vi "Elevator - State Exit.vi"(8 "error in (no error)":errorcluster, 11 "View Model":T1) -> (0 "error out":errorcluster, 3 "View Model":T1)   [LabVIEW 2017]
doc: "Perform actions before finish a specific state."
uses:
  View Model/Controls/View Model.ctl
  Configuration/Controls/Config Model.ctl
  Configuration/Controls/Config Data.ctl
  Error Handler/Controls/Error Model.ctl
  Error Handler/Controls/Error Data.ctl
  Error Handler/Controls/Error Type.ctl
  View Model/Controls/Shared Model.ctl
  Controls/Elevator Model.ctl
  Controls/Elevator Location.ctl
  Controls/Elevator CMD Data.ctl
  Controls/Elevator Commands.ctl
  Controls/Elevator Overhead.ctl
  Controls/Elevator States.ctl
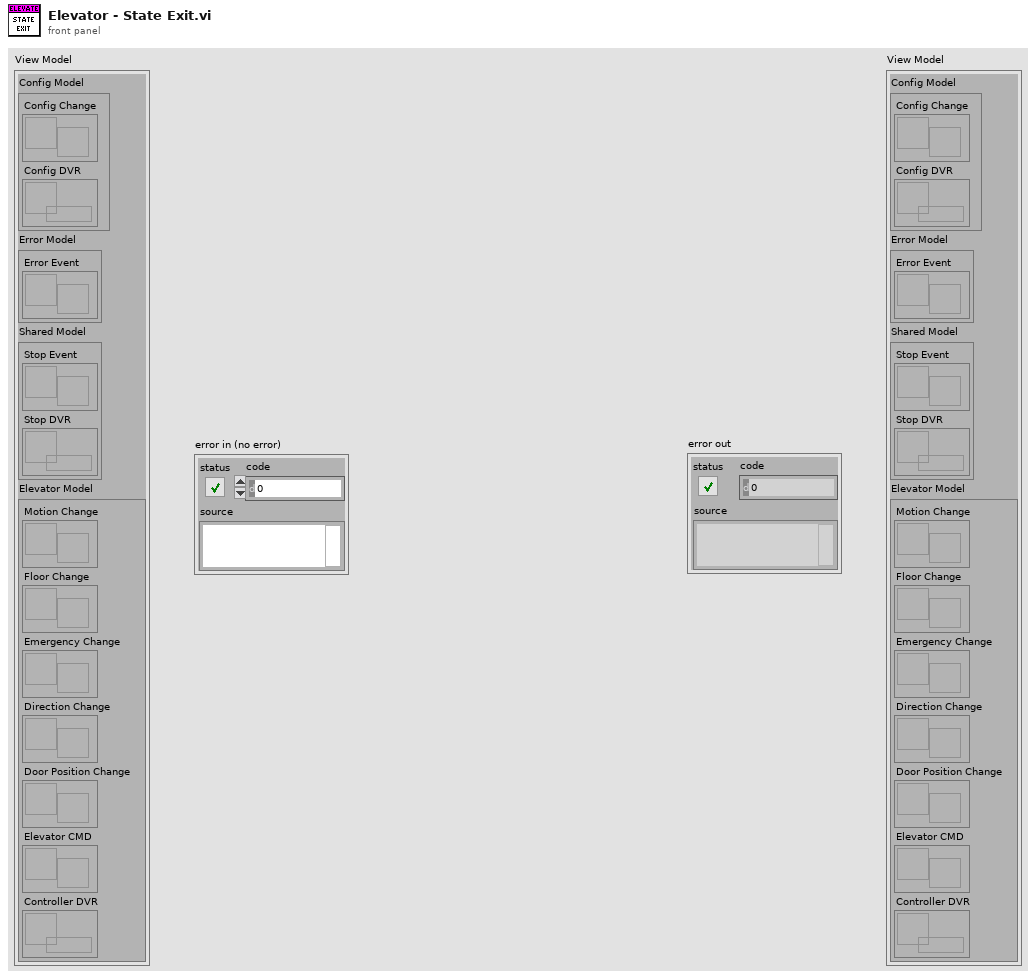
[diagram p1: front panel]
types:
  T1 = typedef "View Model.ctl" = cluster{"Config Model":T2, "Error Model":T3, "Shared Model":T4, "Elevator Model":T5}
  T2 = typedef "Config Model.ctl" = cluster{"Config Change":refnum<user-event>, "Config DVR":refnum<data-value>}
  T3 = typedef "Error Model.ctl" = cluster{"Error Event":refnum<user-event>}
  T4 = typedef "Shared Model.ctl" = cluster{"Stop Event":refnum<user-event>, "Stop DVR":refnum<data-value>}
  T5 = typedef "Elevator Model.ctl" = cluster{"Motion Change":refnum<user-event>, "Floor Change":refnum<user-event>, "Emergency Change":refnum<user-event>, "Direction Change":refnum<user-event>, "Door Position Change":refnum<user-event>, "Elevator CMD":refnum<user-event>, "Controller DVR":refnum<data-value>}
  T6 = typedef "Elevator States.ctl" = enum16{"Initial", "Wait for 1st Request", "Start and Move", "Analysis", "Continue Travel", "Stop at Floor", "Open and Close Door", "No Request", "Emergency", "Terminate"}
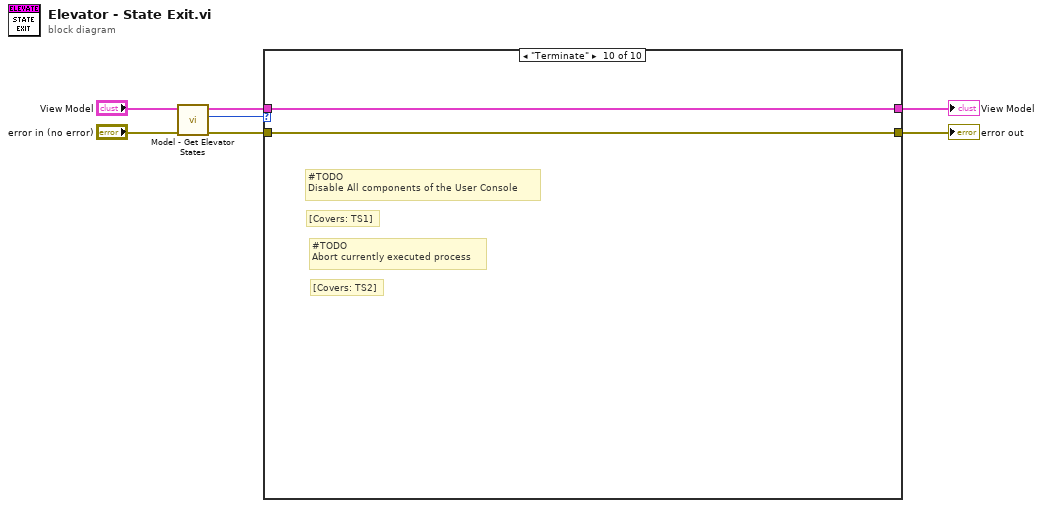
[diagram p0: block diagram]
diagram:
  n1 = call "Model - Get Elevator States.vi"("error in (no error)"="error in (no error)", "View Model"="View Model") -> ("error out"=w3:errorcluster, "Elevator State"=w5:T6, "View Model"=w4:T1)  [unwired: 6 in, 1 out]
  n2 = case shown="\"Terminate\"" w5 {
    tunnel: w4 -> [w9 w11 w13 w15 w17 w19 w21 w23 w25 w27]
    tunnel: w3 -> [w8 w10 w12 w14 w16 w18 w20 w22 w24 w26]
    tunnel: [w9 w11 w13 w15 w17 w19 w21 w23 w25 w27] -> w2
    tunnel: [w8 w10 w12 w14 w16 w18 w20 w22 w24 w26] -> w1
    frame "Initial", Default {
    }
    frame "Wait for 1st Request" {
    }
    frame "Start and Move" {
      # "[Covers: CT1B]"
      # "[Covers: SS4B]"
      # "If time has elapsed, stop elevator. Update floor position"
    }
    frame "Analysis" {
      # "[Covers: AS2C]"
      # "[Covers: AS2B]"
      # "[Covers: AS2A]"
      # "[Covers: AS2]"
      # "[Covers: AS1]"
      # "Handles all analysis"
    }
    frame "Continue Travel" {
    }
    frame "Stop at Floor" {
      # "[Covers: RF2]"
      # "[Covers: RF1]"
      # "#TODO\nTurn off Floor Selection & Elevator call controls\nfor current floor and direction"
      # "[Covers: RF3]"
      # "Transition to door open/close"
    }
    frame "Open and Close Door" {
      # "[Covers: OC7]"
      # "Transition to initial state"
      # "[Covers: OC3B]"
      # "If open door timer <=0, go to close state"
    }
    frame "No Request" {
      # "[Covers: NR1A]"
      # "If inactivity timer <=0, transition to start move with 1st floor as destination"
    }
    frame "Emergency" {
    }
    frame "Terminate" {
      # "[Covers: TS2]"
      # "#TODO\nAbort currently executed process"
      # "[Covers: TS1]"
      # "#TODO\nDisable All components of the User Console"
    }
  }
  "View Model" <- w2
  "error out" <- w1
